vi "Initialize Attributes.vi"(8 "error in (no error)":errorcluster, 10 "Attribute Data":variant, 11 "CS++DIM-Server in":refnum<class "CS++DIM-Server.lvclass">) -> (0 "error out":errorcluster, 2 "Found?":bool, 3 "CS++DIM-Server out":refnum<class "CS++DIM-Server.lvclass">)   [LabVIEW 2016, in "CS++DIM-Server.lvlib" / "CS++DIM-Server.lvclass"]
doc: "Initialize object attribute.\n\nUnique resources should be allocated elsewhere!"
uses:
  CS++DIM-Server.lvclass
  CS++DIM-Server.lvclass/CS++DIM-Server.ctl
  CSPP_Core/Actors/CS++BaseActor/CS++BaseActor.lvclass
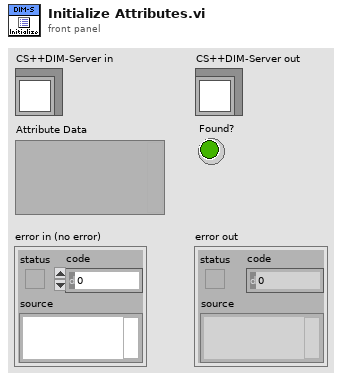
[diagram p1: front panel]
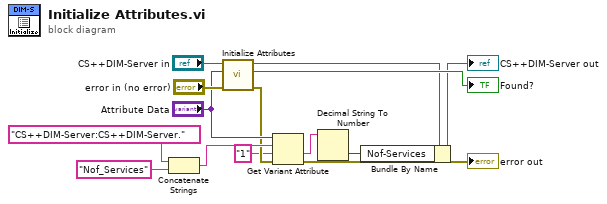
[diagram p0: block diagram]
diagram:
  n1 = Concatenate Strings("CS++DIM-Server:CS++DIM-Server.", "Nof_Services" ("string")) -> (w10:string)
  n2 = call-parent "Initialize Attributes.vi"("error in (no error)"="error in (no error)", "Attribute Data"="Attribute Data", "CS++BaseActor in"="CS++DIM-Server in") -> ("error out"=w7:errorcluster, "Found?"=→"Found?":bool, "CS++BaseActor out"=w5:refnum<class "CS++DIM-Server.lvclass">)  [unwired: 6 in]
  n3 = Get Variant Attribute(Variant="Attribute Data", name=w10, default value (empty Variant)="1" ("string"), error in=w7) -> (value=w2:string, error out=→"error out":errorcluster)  [unwired: 2 out]
  n4 = Decimal String To Number(string=w2) -> (number=w1:i32)  [unwired: 2 in, 1 out]
  n5 = Bundle By Name(cluster=w5, "Nof-Services"=w1) -> (→"CS++DIM-Server out":refnum<class "CS++DIM-Server.lvclass">)
